vi "Sep_Bool.vi"(3 "Relay_Channel_Write":T2 {"Relay_CH_Array"."OUTPUT_Relay_Channels" items=["CONN_SUPPLY_%d_FCT", "HB_CONN_%d_FCT", "L_IND_CONN_%d_FCT", "R_IND_CONN_%d_FCT", "SW1_%d_FCT", "SW2_%d_FCT", "CAN_H_%d_FCT", "CAN_L_%d_FCT", "CYLINDER_ON/OFF_%d_FCT", "SPARE_1_%d_FCT", "SPARE_2_%d_FCT", "Tower Red", "Tower Amber", "Tower Green", "Tower Buzzer", "SLIMRELAY_DUT%d_FCT", "GND_DMM_%d_EOL", "CAN_H_RES_%d_EOL", "CAN_L_RES_%d_EOL", "L_IND_RES_%d_EOL", "R_IND_RES_%d_EOL", "HB_CONN_DMM_%d_EOL", "14V_RES_%d_EOL", "CAN_L_(DMM-)_%d_EOL", "CAN_H_%d_EOL", "CAN_L_%d_EOL", "14V_%d_EOL", "GND_%d_EOL", "HB_CONN_%d_EOL", "L_IND_%d_EOL", "R_IND_%d_EOL", "CYLINDER_DUT_%d_EOL", "CYL_PB_1_%d_EOL", "CYL_PB_2_%d_EOL", "DUT_PASS_%d_EOL", "DUT_FAIL_%d_EOL", "SPARE1_%d_EOL", "Tower Red_EOL", "Tower Amber_EOL", "Tower Green_EOL", "Tower Buzzer_EOL"]}) -> (0 "DO_Bool":bool[](array[boolean]), 1 "DO_Enum":T1[](array[typedef]))   [LabVIEW 2024, in "ADAM_DI.lvlib"]
uses:
  ADAM_DI.lvlib
  Relay_Channel_Write.ctl
  Settings/support/Common_plc_DOs.ctl
  Relay_Enum_OUT.ctl
  Settings/Setting_Screen.lvlib
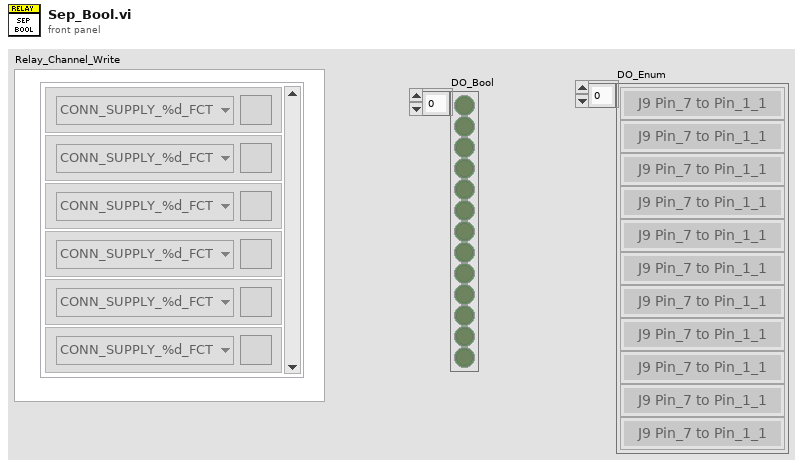
[diagram p1: front panel]
types:
  T1 = typedef "ADAM_DI.lvlib/Relay_Enum_OUT.ctl" = enum16{"J9 Pin_8 to Pin_1_1", "J9 Pin_8 to Pin_1_2", "J9 Pin_7 to Pin_1_1", "J9 Pin_7 to Pin_1_2", "J9 Pin_8 to Pin_7_1", "J9 Pin_8 to Pin_7_2", "J9 Pin_5 to Pin_1_1", "J9 Pin_5 to Pin_1_2", "J9 Pin_6 to Pin_1_1", "J9 Pin_6 to Pin_1_2", "J9 Pin_4 to Pin_1_1", "J9 Pin_4 to Pin_1_2", "J9 Pin_3 to Pin_1_1", "J9 Pin_3 to Pin_1_2", "PS(GND) to Pin1_1 J9", "PS(GND) to Pin1_2 J9", "PS(+14V) to Pin_3_1", "PS(+14V) to Pin_3_2", "PS(+12V) to Pin_4_1_ J9", "PS(+12V) to Pin_4_2_ J9", "PS(+12V) to Pin_5_1 J9", "PS(+12V) to Pin_5_2 J9", "PS(+12V) to Pin_6_1 J9", "PS(+12V) to Pin_6_2 J9", "Tower Amber", "Tower Red", "Tower Green", "Tower Buzzer", "PS(GND) to TP3_1", "PS(GND) to TP3_2", "PS(+14V) to TP19_1", "PS(+14V) to TP19_2", "PS(+12V) to TP33_1", "PS(+12V) to TP33_2", "PS(+12V) to TP38_1", "PS(+12V) to TP38_2", "PS(+12V) to TP40_1", "PS(+12V) to TP40_2", "TP19 (+14V) to TP3 (GND)_1", "TP19 (+14V) to TP3 (GND)_2", "TP1 (+14V) to TP3 (GND)_1", "TP1 (+14V) to TP3 (GND)_2", "TP2 (+5V) to TP3 (GND)_1", "TP2 (+5V) to TP3 (GND)_2", "TP6 (+14V) to TP9 (GND)_1", "TP6 (+14V) to TP9 (GND)_2", "TP7 (+3V8) to TP9 (GND)_1", "TP7 (+3V8) to TP9 (GND)_2", "TP11 (+14V) to TP13 (GND)_1", "TP11 (+14V) to TP13 (GND)_2", "TP12 (+3V) to TP13 (GND)_1", "TP12 (+3V) to TP13 (GND)_2", "TP5 (+3V3) to TP8 (GND)_1", "TP5 (+3V3) to TP8 (GND)_2", "TP48 (CAN_H) to TP3 (GND)_1", "TP48 (CAN_H) to TP3 (GND)_2", "TP41 (CAN_L) to TP3 (GND)_1", "TP41 (CAN_L) to TP3 (GND)_2", "TP48 (CAN_H) to TP41 (CAN_L)_1", "TP48 (CAN_H) to TP41 (CAN_L)_2", "TP38 (L_IND) to TP3 (GND)_1", "TP38 (L_IND) to TP3 (GND)_2", "TP40 (R_IND) to TP3 (GND)_1", "TP40 (R_IND) to TP3 (GND)_2", "TP33 (HB_CON) to TP3 (GND)_1", "TP33 (HB_CON) to TP3 (GND)_2", "TP19 (+14V) to TP34 (Q19-G)_1", "TP19 (+14V) to TP34 (Q19-G)_2", "TP55 (SW1) to TP3 (GND)_1", "TP55 (SW1) to TP3 (GND)_2", "TP56 (SW2) to TP3 (GND)_1", "TP56 (SW2) to TP3 (GND)_2", "TP66 WRT TP3 (GND)_1", "TP66 WRT TP3 (GND)_2", "TP19 WRT TP3_1", "TP19 WRT TP3_2", "TP1 WRT TP3_1", "TP1 WRT TP3_2", "TP2 WRT TP3_1", "TP2 WRT TP3_2", "TP7 WRT TP9_1", "TP7 WRT TP9_2", "TP12 WRT TP13_1", "TP12 WRT TP13_2", "TP5 WRT TP8_1", "TP5 WRT TP8_2", "TP22 WRT TP3_1", "TP22 WRT TP3_2", "TP52 WRT TP3(GND)_1", "TP52 WRT TP3(GND)_2", "TP50 WRT TP3(GND)_1", "TP50 WRT TP3(GND)_2", "TP51 WRT TP3(GND)_1", "TP51 WRT TP3(GND)_2"}
  T2 = typedef "ADAM_DI.lvlib/Relay_Channel_Write.ctl" = cluster{"Relay_CH_Array":cluster{"OUTPUT_Relay_Channels":T3, "On/Off":bool}[]}
  T3 = typedef "Setting_Screen.lvlib/Common_plc_DOs.ctl" = u16
  T4 = cluster{"OUTPUT_Relay_Channels":T3, "On/Off":bool}[]
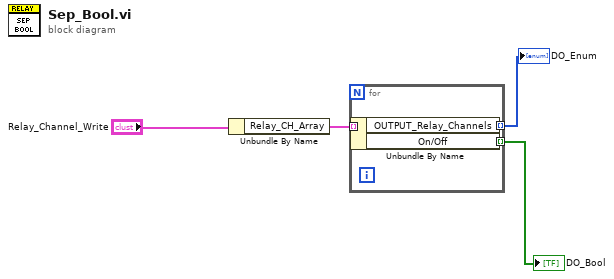
[diagram p0: block diagram]
diagram:
  n1 = Unbundle By Name("Relay_Channel_Write") -> ("Relay_CH_Array"=w3:T4)
  n2 = for {
    tunnel: w3 -> [w7] mode=indexing
    tunnel: [w6] -> w2 mode=indexing
    tunnel: [w5] -> w1 mode=indexing
    n3 = Unbundle By Name(w7) -> ("OUTPUT_Relay_Channels"=w6:T3, "On/Off"=w5:bool)
  }
  "DO_Enum" <- w2
  "DO_Bool" <- w1
